vi "test ini.vi"() -> ()   [LabVIEW 2019]
uses:
  setpoints.ctl
  backwash.ctl
  coag.ctl
  model type.ctl
  file paths.ctl
  ini.ctl
panel:
  in  "setpoints":T1={"graph data interval (s)"=5.0, "sludge flow [L/s]"=0.001, "plant flow [L/s]"=0.5, "Plant Flow PID "={"proportional gain (Kc)"=10.0, "integral time (Ti, min)"=0.4, "derivative time (Td, min)"=0.0}, "Sludge PID "={"proportional gain (Kc)"=0.07, "integral time (Ti, min)"=1.0, "derivative time (Td, min)"=0.01}, "backwash"={"Filtered quality target [NTU]"=0.2, "min filtration time [s]"=3600.0, "Ripen time [s]"=600.0}, "Coagulant"={"flocculator volume (L)"=66.81, "clarifier volume (L)"=2.0, "dose updates per HRT"=10, "target clarified turbidity (NTU)"=0.6, "Coagulant mode"=enum."manual", "Coag dose [mg/L]"=5.5, "pump mL/rev"=0.255, "clarifier flow [L/s]"=0.0033, "min Coag dose [mg/L]"=2.0, "max Coag dose [mg/L]"=6.0, "Steps"=3, "HRT response delay"=2, "Ku*"=1.0, "DOM coag demand [mg/L]"=0.0, "min DOM coag demand [mg/L]"=0.0, "max DOM coag demand [mg/L]"=0.0}} {"Coagulant"."max DOM coag demand [mg/L]" min=0.0 max=20.0 step=0.1; "Coagulant"."min DOM coag demand [mg/L]" min=0.0 max=10.0 step=0.1; "Coagulant"."DOM coag demand [mg/L]" min=0.0 max=20.0 step=0.1; "Coagulant"."HRT response delay" min=1 max=10 step=1; "Coagulant"."Steps" min=3 step=1; "Coagulant"."clarifier flow [L/s]" min=0.0001 max=1.0 step=0.0001; "Coagulant"."target clarified turbidity (NTU)" min=0.1 max=5.0 step=0.01; "Coagulant"."dose updates per HRT" min=1 max=100 step=1; "Sludge PID"."derivative time (Td, min)" format="%.3f"; "Sludge PID"."integral time (Ti, min)" format="%.3f"; "Sludge PID"."proportional gain (Kc)" format="%.3f"; "Plant Flow PID"."derivative time (Td, min)" format="%.3f"; "Plant Flow PID"."integral time (Ti, min)" format="%.3f"; "Plant Flow PID"."proportional gain (Kc)" format="%.3f"; "plant flow [L/s]" min=0.05 max=1.0 step=0.05; "sludge flow [L/s]" min=0.0 max=0.05 step=0.001; "graph data interval (s)" min=1 max=1000 step=1}
  out "Setpoints out":T1={"graph data interval (s)"=100.0, "sludge flow [L/s]"=0.0, "plant flow [L/s]"=0.0, "Plant Flow PID "={"proportional gain (Kc)"=0.05, "integral time (Ti, min)"=1.0, "derivative time (Td, min)"=0.01}, "Sludge PID "={"proportional gain (Kc)"=0.07, "integral time (Ti, min)"=1.0, "derivative time (Td, min)"=0.01}, "backwash"={"Filtered quality target [NTU]"=0.3, "min filtration time [s]"=600.0, "Ripen time [s]"=600.0}, "Coagulant"={"flocculator volume (L)"=0.0, "clarifier volume (L)"=0.0, "dose updates per HRT"=100, "target clarified turbidity (NTU)"=0.3, "Coagulant mode"=enum."manual", "Coag dose [mg/L]"=0.0, "pump mL/rev"=0.0, "clarifier flow [L/s]"=0.5, "min Coag dose [mg/L]"=0.0, "max Coag dose [mg/L]"=0.0, "Steps"=3, "HRT response delay"=1, "Ku*"=1.0, "DOM coag demand [mg/L]"=0.0, "min DOM coag demand [mg/L]"=0.0, "max DOM coag demand [mg/L]"=0.0}} {"Coagulant"."max DOM coag demand [mg/L]" min=0.0 max=20.0 step=0.1; "Coagulant"."min DOM coag demand [mg/L]" min=0.0 max=10.0 step=0.1; "Coagulant"."DOM coag demand [mg/L]" min=0.0 max=20.0 step=0.1; "Coagulant"."HRT response delay" min=1 max=10 step=1; "Coagulant"."Steps" min=3 step=1; "Coagulant"."clarifier flow [L/s]" min=0.0001 max=1.0 step=0.0001; "Coagulant"."target clarified turbidity (NTU)" min=0.1 max=5.0 step=0.01; "Coagulant"."dose updates per HRT" min=1 max=100 step=1; "Sludge PID"."derivative time (Td, min)" format="%.3f"; "Sludge PID"."integral time (Ti, min)" format="%.3f"; "Sludge PID"."proportional gain (Kc)" format="%.3f"; "Plant Flow PID"."derivative time (Td, min)" format="%.3f"; "Plant Flow PID"."integral time (Ti, min)" format="%.3f"; "Plant Flow PID"."proportional gain (Kc)" format="%.3f"; "plant flow [L/s]" min=0.05 max=1.0 step=0.05; "sludge flow [L/s]" min=0.0 max=0.05 step=0.001; "graph data interval (s)" min=1 max=1000 step=1}
  in  "stop":bool
  in  "write":bool
  in  "read":bool
  # "ramp controls"
  # "min"
  # "max"
  # "min"
  # "max"
  # "ramp controls"
  # "min"
  # "max"
  # "min"
  # "max"
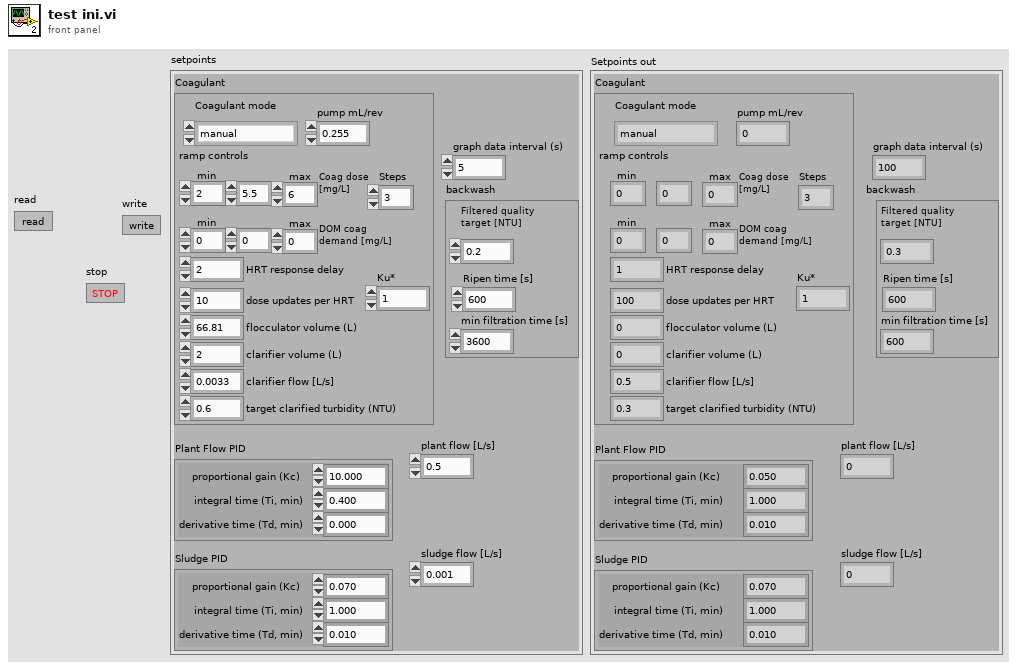
[diagram p1: front panel]
types:
  T1 = typedef "setpoints.ctl" = cluster{"graph data interval (s)":sgl, "sludge flow [L/s]":dbl, "plant flow [L/s]":dbl, "Plant Flow PID ":cluster{"proportional gain (Kc)":dbl, "integral time (Ti, min)":dbl, "derivative time (Td, min)":dbl}, "Sludge PID ":cluster{"proportional gain (Kc)":dbl, "integral time (Ti, min)":dbl, "derivative time (Td, min)":dbl}, "backwash":T2, "Coagulant":T3}
  T2 = typedef "backwash.ctl" = cluster{"Filtered quality target [NTU]":dbl, "min filtration time [s]":dbl, "Ripen time [s]":dbl}
  T3 = typedef "coag.ctl" = cluster{"flocculator volume (L)":dbl, "clarifier volume (L)":dbl, "dose updates per HRT":u16, "target clarified turbidity (NTU)":dbl, "Coagulant mode":T4, "Coag dose [mg/L]":dbl, "pump mL/rev":dbl, "clarifier flow [L/s]":dbl, "min Coag dose [mg/L]":dbl, "max Coag dose [mg/L]":dbl, "Steps":u16, "HRT response delay":u32, "Ku*":dbl, "DOM coag demand [mg/L]":dbl, "min DOM coag demand [mg/L]":dbl, "max DOM coag demand [mg/L]":dbl}
  T4 = typedef "model type.ctl" = enum16{"manual", "ramp", "simple corrector"}
  T5 = typedef "ini.ctl" = enum16{"write", "read"}
  T6 = typedef "file paths.ctl" = enum16{"read paths", "close"}
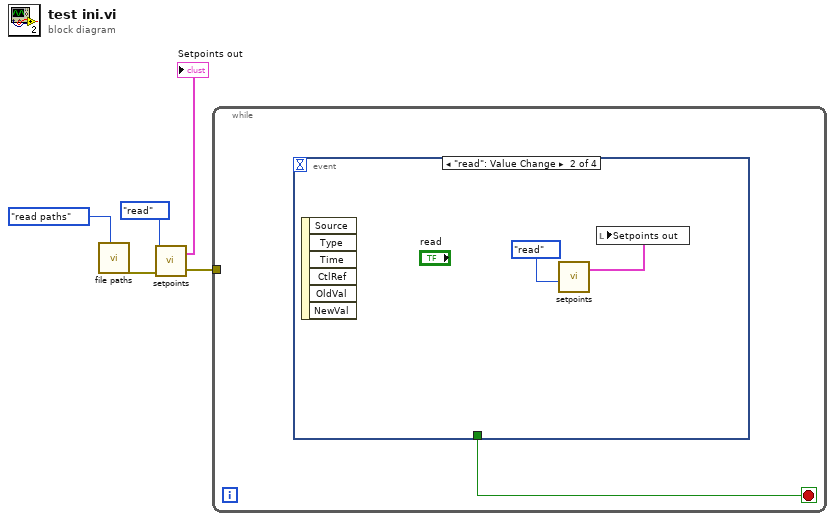
[diagram p0: block diagram]
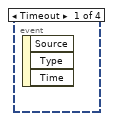
[diagram p2: hidden frame]
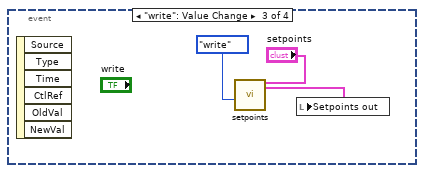
[diagram p3: hidden frame]
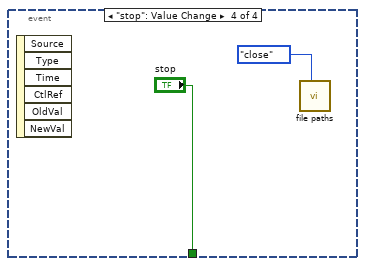
[diagram p4: hidden frame]
diagram:
  n1 = call "file paths.vi"("file path control"=file_paths."read paths") -> ("error out"=w4:errorcluster)  [unwired: 7 in, 3 out]
  n2 = call "setpoints.vi"("error in (no error)"=w4, "ini"=ini."read") -> ("error out"=w1:errorcluster, "Setpoints out"=→"Setpoints out":T1)  [unwired: 8 in]
  n3 = while {
    tunnel: w1 -> [_]
    stop <- w6 stop-if-true
    n4 = event shown="[1] \"read\": Value Change" {
      selector: _ -> [_ _ _ _]
      dyn-events: _ -> [_ _ _ _]
      timeout: _ -> [_ _ _ _]
      tunnel: [_ _ _ "stop"] -> w6
      event Timeout {
        n5 = event-data() -> ()  [unwired: 1 in, 3 out]
      }
      event "read": Value Change {
        n6 = event-data() -> ()  [unwired: 1 in, 6 out]
        n7 = call "setpoints.vi"("ini"=ini."read") -> ("Setpoints out"=w7:T1)  [unwired: 9 in, 1 out]
        n8 = local write "Setpoints out"(w7) -> ()
      }
      event "write": Value Change {
        n9 = event-data() -> ()  [unwired: 1 in, 6 out]
        n10 = call "setpoints.vi"("setpoints"="setpoints", "ini"=ini."write") -> ("Setpoints out"=w9:T1)  [unwired: 8 in, 1 out]
        n11 = local write "Setpoints out"(w9) -> ()
      }
      event "stop": Value Change {
        n12 = event-data() -> ()  [unwired: 1 in, 6 out]
        n13 = call "file paths.vi"("file path control"=file_paths."close") -> ()  [unwired: 7 in, 4 out]
      }
    }
  }
